vi "ConvertHexSetpointToNumeric.vi"(11 "Hex Setpoint":string="0044C") -> (3 "Numeric Setpoint (C)":dbl format="%.1f")   [LabVIEW 2012, in "Omega-CSi32.lvlib"]
uses:
  Omega-CSi32.lvlib
panel:
  out "substring":string
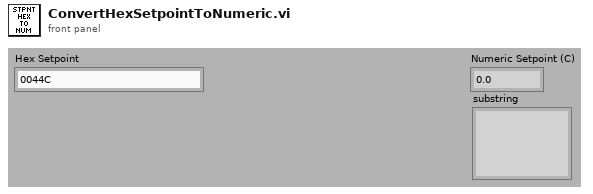
[diagram p1: front panel]
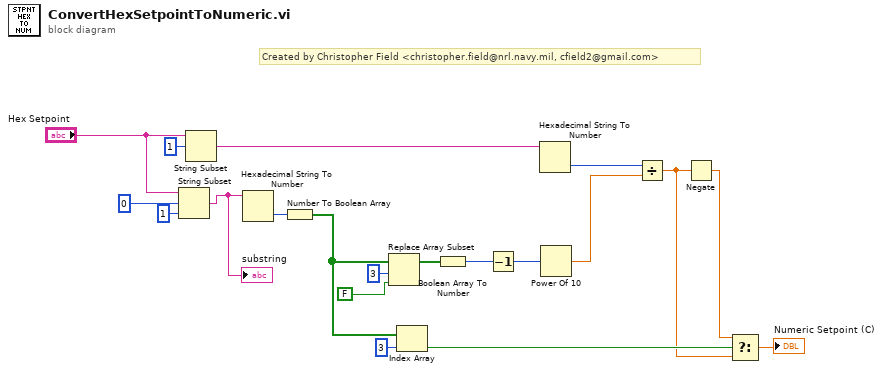
[diagram p0: block diagram]
diagram:
  # "Created by Christopher Field <christopher.field@nrl.navy.mil, cfield2@gmail.com>"
  n1 = String Subset(string="Hex Setpoint", offset (0)=0, length (rest)=1 ("length (rest)")) -> (substring=w4:string)
  "substring" <- w4
  n2 = String Subset(string="Hex Setpoint", offset (0)=1) -> (substring=w19:string)  [unwired: 1 in]
  n3 = Hexadecimal String To Number(string=w4) -> (number=w18:u32)  [unwired: 2 in, 1 out]
  n4 = Number To Boolean Array(number=w18) -> (Boolean array=w14:bool[])
  n5 = Replace Array Subset(array=w14, new element=FALSE ("new element/subarray"), index=3) -> (w15:bool[])
  n6 = Index Array(array=w14, index=3) -> (element=w12:bool)
  n7 = Boolean Array To Number(Boolean array=w15) -> (number=w11:u32)
  n8 = Decrement(x=w11) -> (x-1=w10:u32)
  n9 = Hexadecimal String To Number(string=w19) -> (number=w9:u32)  [unwired: 2 in, 1 out]
  n10 = Power Of 10(x=w10) -> (10^x=w8:dbl)
  n11 = Divide(x=w9, y=w8) -> (x/y=w6:dbl)
  n12 = Negate(x=w6) -> (-x=w7:dbl)
  n13 = Select(t=w7, s=w12, f=w6) -> (s? t:f=→"Numeric Setpoint (C)":dbl)
